vi "SynapseAPI-Get Parameter Names.vi"(0 "URL":string="http://localhost:24414", 7 "gizmo":string, 11 "error in (no error)":errorcluster) -> (8 "parameters":string[](array[string]), 15 "error out":errorcluster)   [LabVIEW 2020]
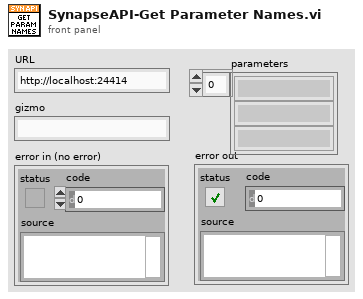
[diagram p1: front panel]
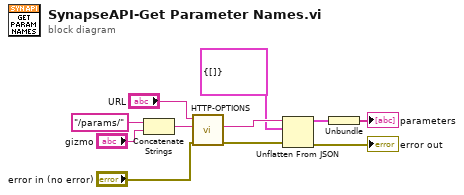
[diagram p0: block diagram]
diagram:
  n1 = Concatenate Strings("/params/", "gizmo") -> (w2:string)
  n2 = call "HTTP-OPTIONS.vi"("error in (no error)"="error in (no error)", "req"=w2, "URL"="URL") -> ("error out"=w8:errorcluster, "body"=w7:string)  [unwired: 6 in, 1 out]
  n3 = Unflatten From JSON(JSON string=w7, type and defaults=cluster{"parameters":string[]} {"parameters"=[]}, error in (no error)=w8) -> (value=w4:cluster{"parameters":string[]}, error out=→"error out":errorcluster)  [unwired: 4 in]
  n4 = Unbundle(w4) -> ("parameters"=→"parameters":string[])
